vi "FlatToRichrouteguide_RouteSummary.vi"(5 "OutputClusterType":T1, 11 "InputCluster":T2) -> (3 "OutputCluster":T1)   [LabVIEW 2019, in "route_guide_client.lvlib"]
uses:
  route_guide_client.lvlib
  routeguide_RouteSummary_Flat.ctl
  routeguide_RouteSummary.ctl
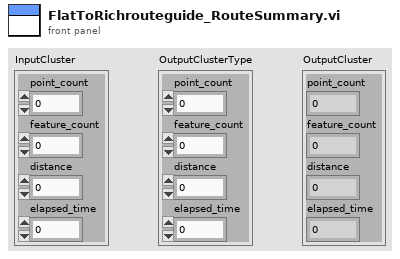
[diagram p1: front panel]
types:
  T1 = typedef "route_guide_client.lvlib/routeguide_RouteSummary.ctl" = cluster{"point_count":i32, "feature_count":i32, "distance":i32, "elapsed_time":i32}
  T2 = typedef "route_guide_client.lvlib/routeguide_RouteSummary_Flat.ctl" = cluster{"point_count":i32, "feature_count":i32, "distance":i32, "elapsed_time":i32}
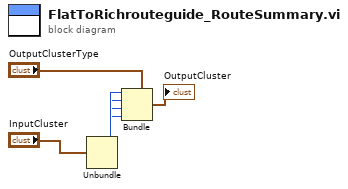
[diagram p0: block diagram]
diagram:
  n1 = Unbundle "Unbundle"("InputCluster") -> ("point_count"=w4:i32, "feature_count"=w3:i32, "distance"=w2:i32, "elapsed_time"=w1:i32)
  n2 = Bundle "Bundle"(cluster="OutputClusterType", "point_count"=w4, "feature_count"=w3, "distance"=w2, "elapsed_time"=w1) -> (→"OutputCluster":T1)
